vi "histeresis.vi"(9 "paso":dbl, 10 "fin":dbl, 11 "inicio":dbl) -> (2 "Array":dbl[](array[numeric]))   [LabVIEW 2016]
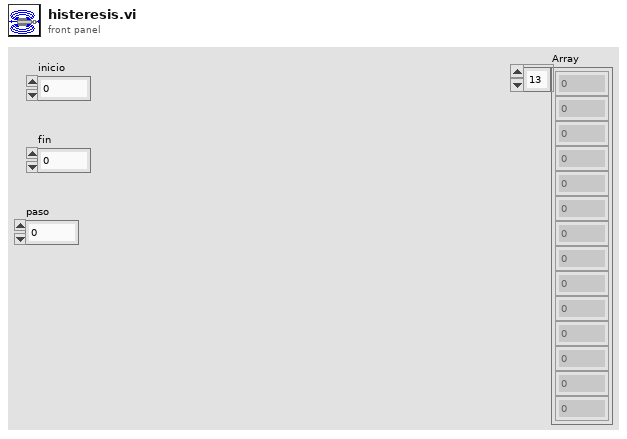
[diagram p1: front panel]
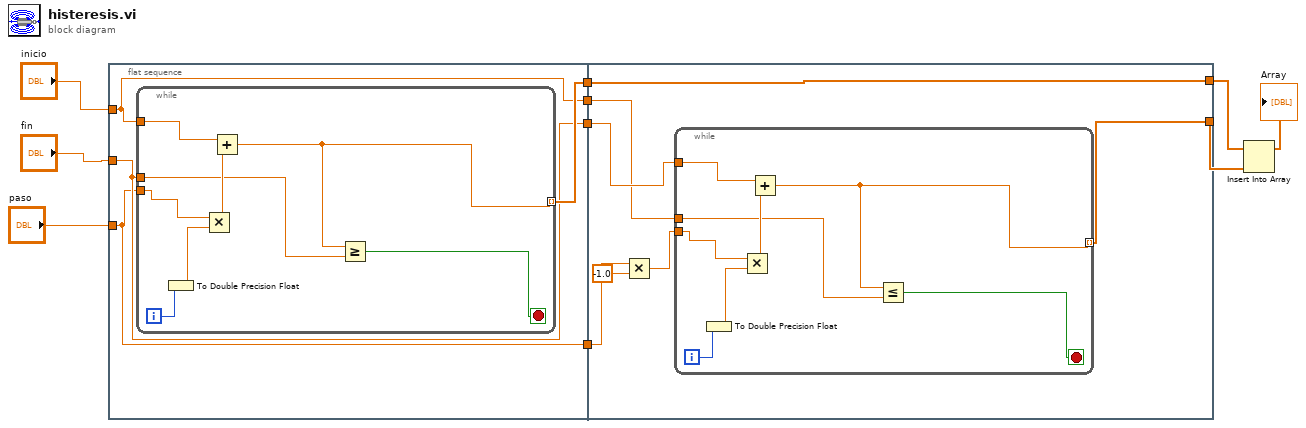
[diagram p0: block diagram]
diagram:
  n1 = flat-sequence {
    tunnel: "inicio" -> [w13]
    tunnel: "fin" -> [w12]
    tunnel: "paso" -> [w11]
    tunnel: [w14] -> w7
    tunnel: [w13] -> w6
    tunnel: [w12] -> w5
    tunnel: [w11] -> w4
    tunnel: [w29] -> w2
    tunnel: w7 -> [w29]
    tunnel: w6 -> [w23]
    tunnel: w5 -> [w24]
    tunnel: w4 -> [w27]
    tunnel: [w25] -> w1
    frame #0 {
      n2 = while {
        tunnel: w13 -> [w22]
        tunnel: w11 -> [w19]
        tunnel: [w17] -> w14 mode=indexing
        tunnel: w12 -> [w16]
        i -> [w21]
        stop <- w15 stop-if-true
        n3 = To Double Precision Float(number=w21) -> (double precision float=w20:dbl)
        n4 = Multiply(x=w19, y=w20) -> (x*y=w18:dbl)
        n5 = Add(x=w22, y=w18) -> (x+y=w17:dbl)
        n6 = Greater Or Equal?(x=w17, y=w16) -> (x >= y?=w15:bool)
      }
    }
    frame #1 {
      n7 = Multiply(x=w27, y=-1.0) -> (x*y=w28:dbl)
      n8 = while {
        tunnel: w24 -> [w37]
        tunnel: w28 -> [w34]
        tunnel: [w32] -> w25 mode=indexing
        tunnel: w23 -> [w31]
        i -> [w36]
        stop <- w30 stop-if-true
        n9 = To Double Precision Float(number=w36) -> (double precision float=w35:dbl)
        n10 = Multiply(x=w34, y=w35) -> (x*y=w33:dbl)
        n11 = Add(x=w37, y=w33) -> (x+y=w32:dbl)
        n12 = Less Or Equal?(x=w32, y=w31) -> (x <= y?=w30:bool)
      }
    }
  }
  n13 = Insert Into Array(array=w2, new element=w1) -> (→"Array":dbl[])  [unwired: 1 in]
